vi "boolToDigitalLevel.vi"(11 "Input":bool) -> (3 "Digital Signal Level":T1)   [LabVIEW 2015]
uses:
  Typedefs/Digital Signal Level.ctl
  Typedefs/ILCBTTypedefs.lvlib
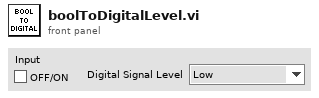
[diagram p1: front panel]
types:
  T1 = typedef "ILCBTTypedefs.lvlib/Digital Signal Level.ctl" = enum16{"Low", "High"}
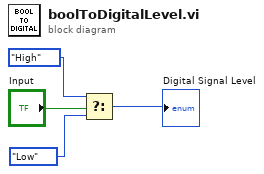
[diagram p0: block diagram]
diagram:
  n1 = Select(t=Digital_Signal_Level."High" ("Digital Signal Level"), s="Input", f=Digital_Signal_Level."Low" ("Digital Signal Level")) -> (s? t:f=→"Digital Signal Level":T1)
